vi "Convert micron to voltage.vi"(8 "error in (no error)":errorcluster, 11 "Piezo in":refnum<class "Piezo.lvclass">) -> (0 "error out":errorcluster, 2 "Output voltage":dbl[unit], 3 "Piezo out":refnum<class "Piezo.lvclass">)   [LabVIEW 2012, in "Piezo.lvclass"]
uses:
  Piezo.lvclass
  Piezo.lvclass/Piezo.ctl
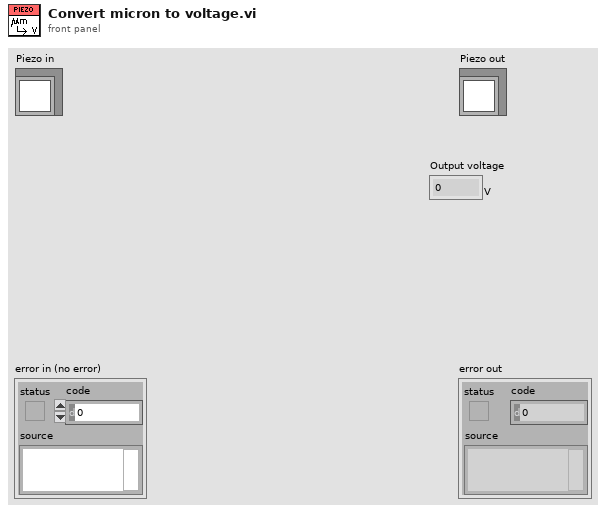
[diagram p1: front panel]
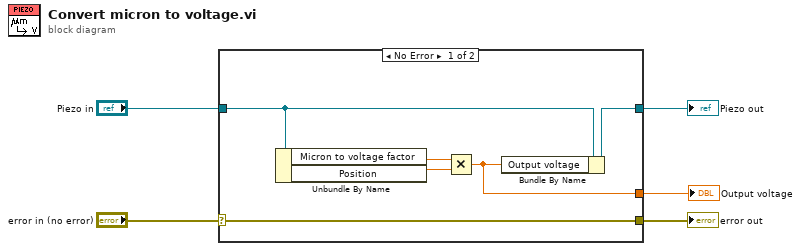
[diagram p0: block diagram]
diagram:
  n1 = case shown="No Error" "error in (no error)" {
    selector: "error in (no error)" -> [w11 w13]
    tunnel: [w11 w13] -> w4
    tunnel: [w7 w12] -> w2
    tunnel: "Piezo in" -> [w8 w12]
    tunnel: [w6 _] -> w1
    frame No Error {
      n2 = Unbundle By Name(w8) -> ("Micron to voltage factor"=w10:dbl[unit], "Position"=w9:dbl[unit])
      n3 = Multiply(x=w10, y=w9) -> (x*y=w6:dbl[unit])
      n4 = Bundle By Name(cluster=w8, "Output voltage"=w6) -> (w7:refnum<class "Piezo.lvclass">)
    }
    frame Error {
    }
  }
  "error out" <- w4
  "Piezo out" <- w2
  "Output voltage" <- w1
